vi "ScanHarmonics Nov21-2018.vi"() -> ()   [LabVIEW 2016]
uses:
  <vilib>/Instr/_visa.llb/VISA Configure Serial Port (Instr).vi
panel:
  out "Current Position 2":string="0\r\n"
  out "Start Time":string
  out "RoiSum":dbl=24008.0
  in  "Main UI":T1(tab)=enum."Collect Data"
  in  "Get Position":bool
  in  "Set Zero Position":bool
  in  "Move to Target":bool
  in  "Arduino USB Port":refnum<visa-resource-name>="COM3"
  in  "Target Motor Position":i32
  out "Current Position":string="0\r\n"
  in  "Reset Arduino":bool
  out "Settings":T2={"Range"=3520, "cftfak"=39321856, "RoiMin"=0, "RoiMax"=3520, "#Regions"=0, "Caluse"=1, "Calpoints"=0, "Param"=0, "Offset"=0, "Xdim"=0, "bitshift"=0, "Active"=1, "Roipreset"=10.0, "dummy1"=0.0, "dummy2"=0.0, "dummy3"=0.0} {"dummy3" format="%.2f"; "dummy2" format="%.2f"; "bitshift" format="%.0x"; "Active" format="%.0x"; "Offset" format="%.0x"; "Param" format="%.0x"; "dummy1" format="%.2f"; "Roipreset" format="%.2f"; "cftfak" format="%.0x"}
  in  "Maximum Scan\nPosition":dbl=3000.0
  out "Harmonics":cluster{"Y":dbl[], "Y":dbl[]}[](graph)=[{"Y"=[200.0, 300.0, 400.0, 500.0, 600.0, 700.0, 800.0, 900.0, 1000.0, 1100.0, 1200.0, 1300.0, 1400.0, 1500.0, 1600.0, 1700.0, 1800.0, 1900.0, 2000.0, 2100.0, 2200.0, 2300.0, 2400.0, 2500.0, 2600.0, 2700.0, 2800.0, 2900.0, 3000.0, 3100.0, 3200.0, 3300.0], "Y"=[0.0, 24008.0, 24008.0, 24008.0, 24008.0, 24008.0, 24008.0, 24008.0, 24008.0, 24008.0, 24008.0, 24008.0, 24008.0, 24008.0, 24008.0, 24008.0, 24008.0, 24008.0, 24008.0, 24008.0, 24008.0, 24008.0, 24008.0, 24008.0, 24008.0, 24008.0, 24008.0, 24008.0, 24008.0, 24008.0, 24008.0, 24008.0]}]
  in  "Start Scan":bool
  out "Spectrum":u32[](graph)
  in  "State":T3(ring)=enum."Move Grating"
  out "Grating Position":i16=3300
  in  "Step Size":i32=100
  in  "Sweeps":i32
  out "CHN Status":T4={"Started"=0, "Maxval"=3001, "Runtime"=0.018000000000000002, "Fifo full"=0.0, "TotalSum"=24008.0, "RoiSum"=24008.0, "Roirate"=0.0, "Sweeps"=3001.0, "Starts"=3001.0, "Dummy"=0.0} {"Dummy" format="%.2f"; "Starts" format="%.2f"; "Sweeps" format="%.2f"; "Roirate" format="%.2f"; "RoiSum" format="%.2f"; "TotalSum" format="%.2f"; "Fifo full" format="%.2f"; "Runtime" format="%.2f"}
  in  "Photoelectron Spectra Destination":path=path "C:/Users/cj09d/Desktop/SpectraTest/Today"
  out "Halt Confirmation":string="OK"
  out "MCSADat Error":i32
  in  "Spectrum #":i32
  out "Arduino Response":string="1600\r\n"
  out "Sent Message":string="M003300#"
  in  "Stop":bool
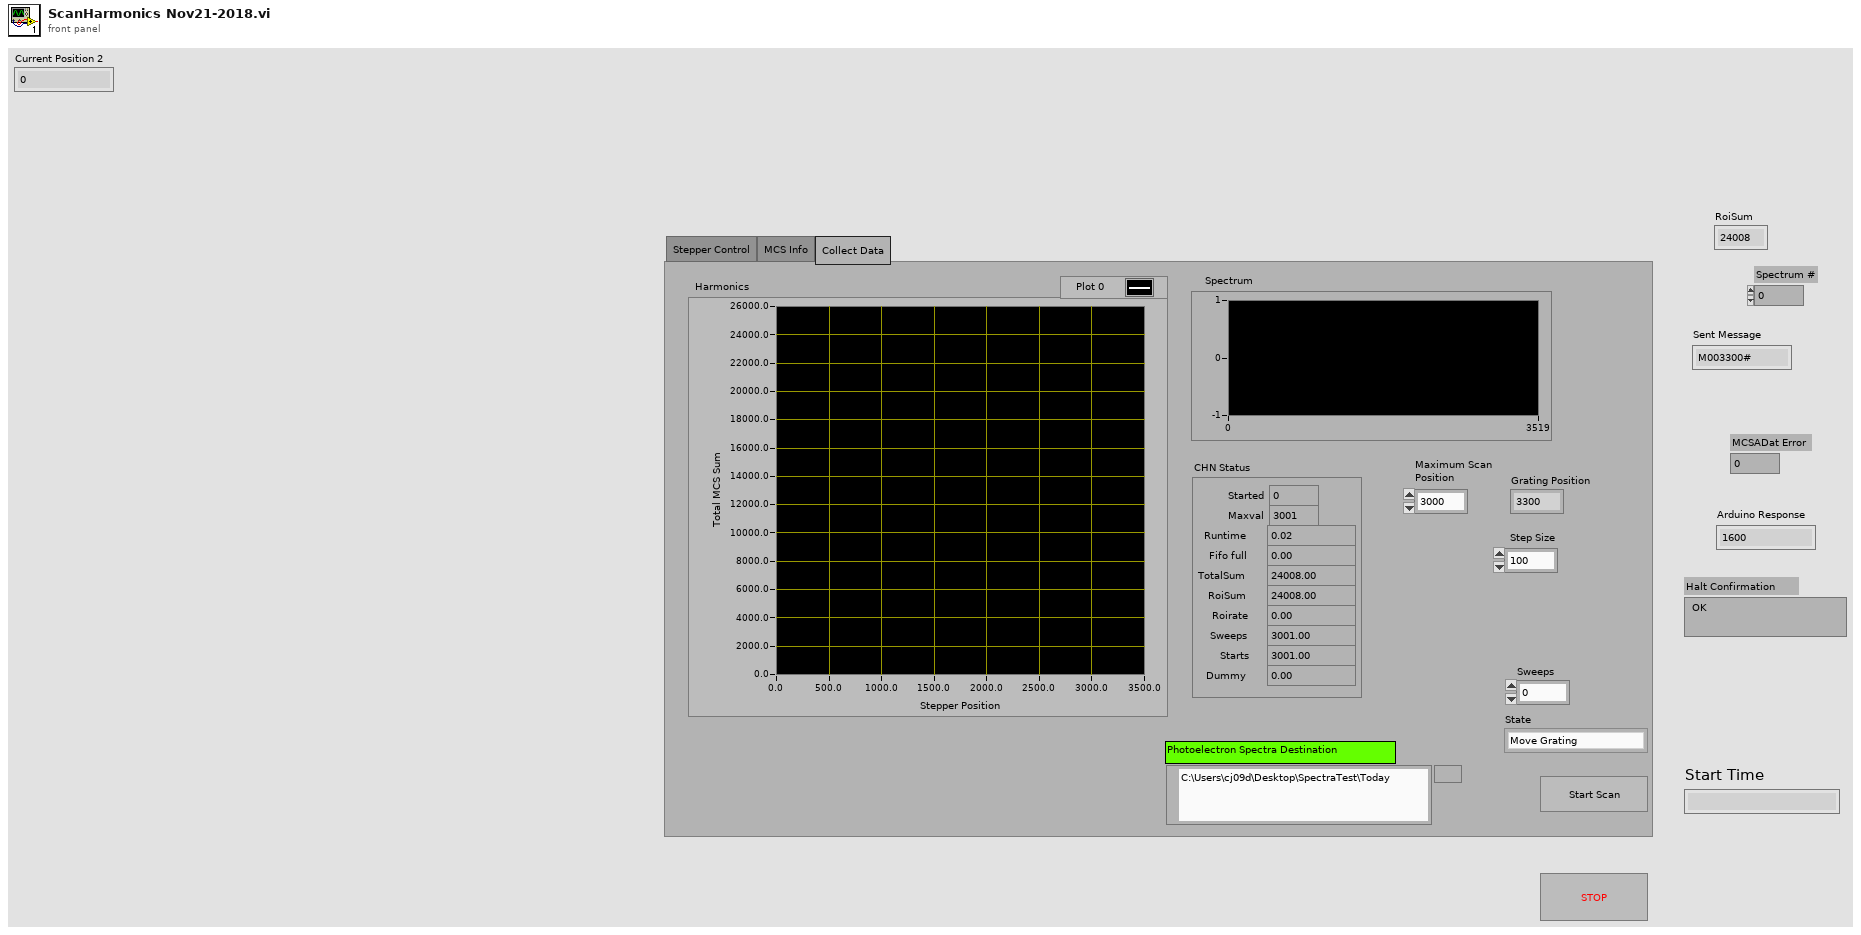
[diagram p1: front panel]
types:
  T1 = enum32{"Stepper Control", "MCS Info", "Collect Data"}
  T2 = cluster{"Range":i32, "cftfak":i32, "RoiMin":i32, "RoiMax":i32, "#Regions":i32, "Caluse":i32, "Calpoints":i32, "Param":i32, "Offset":i32, "Xdim":i32, "bitshift":i32, "Active":i32, "Roipreset":dbl, "dummy1":dbl, "dummy2":dbl, "dummy3":dbl}
  T3 = enum16{"Start", "Move Grating", "Start MCS", "Collect Data", "Stop MCS", "Save Data", "Stop"}
  T4 = cluster{"Started":i32, "Maxval":u32, "Runtime":dbl, "Fifo full":dbl, "TotalSum":dbl, "RoiSum":dbl, "Roirate":dbl, "Sweeps":dbl, "Starts":dbl, "Dummy":dbl}
  T5 = enum16{"open", "replace", "create", "open or create", "replace or create", "replace or create with confirmation"}
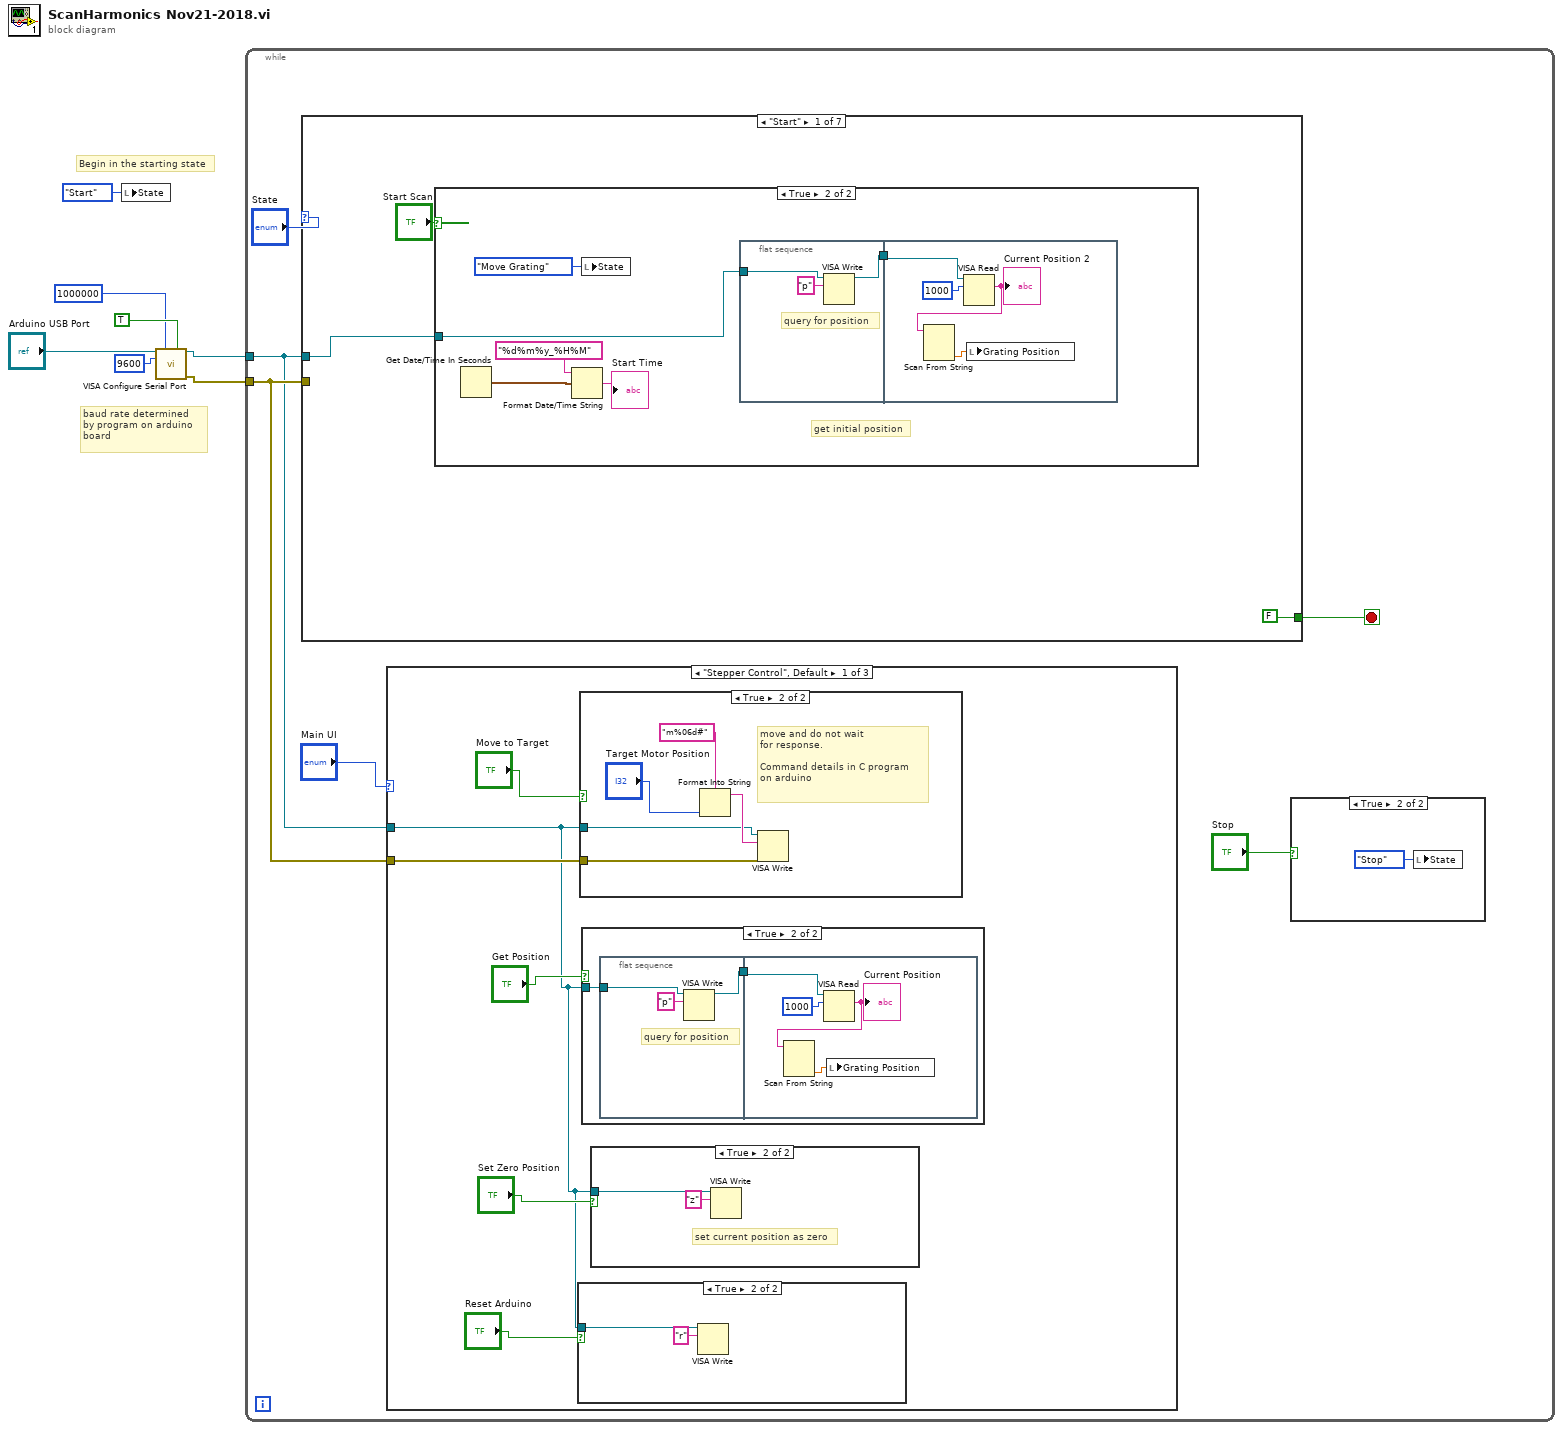
[diagram p0: block diagram]
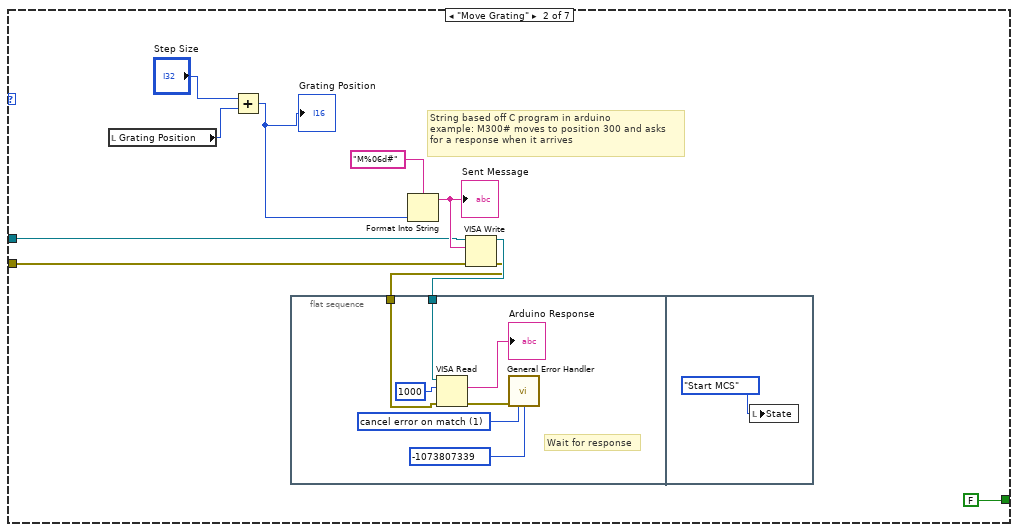
[diagram p10: hidden frame]
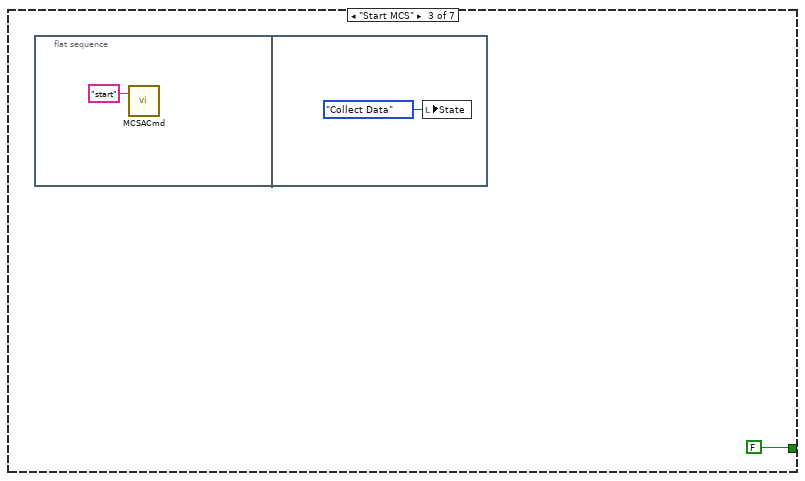
[diagram p11: hidden frame]
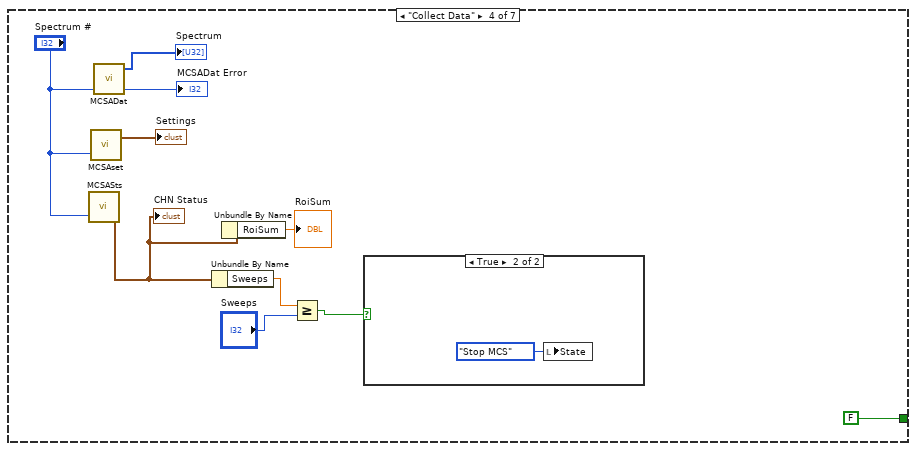
[diagram p12: hidden frame]
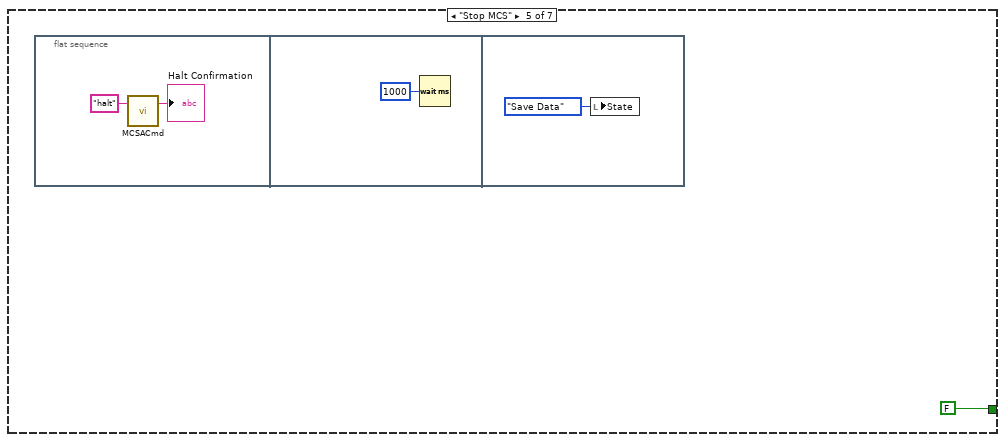
[diagram p14: hidden frame]
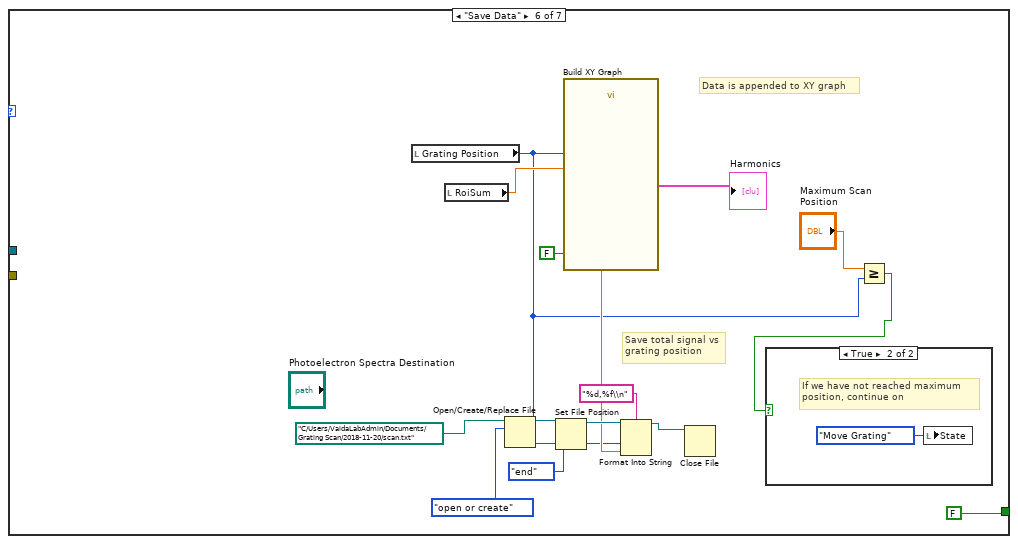
[diagram p15: hidden frame]
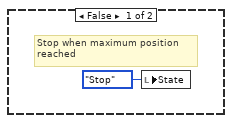
[diagram p16: hidden frame]
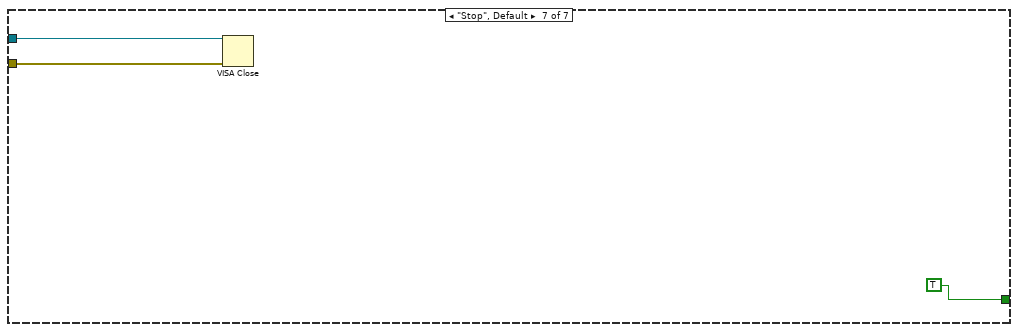
[diagram p17: hidden frame]
diagram:
  # "Begin in the starting state"
  # "baud rate determined\nby program on arduino\nboard"
  n1 = local write "State"(T3."Start" ("State")) -> ()
  n2 = call-poly "VISA Configure Serial Port"("VISA resource name"="Arduino USB Port", "timeout (10sec)"=u32 1000000, "Enable Termination\nChar (T)"=TRUE, "baud rate (9600)"=u32 9600 ("baud rate")) -> ("VISA resource name out"=w1:refnum<visa-resource-name>, "error out"=w2:errorcluster)  [unwired: 6 in, 4 out]
  n3 = while {
    tunnel: w1 -> [w10]
    tunnel: w2 -> [w11]
    stop <- w9 stop-if-true
    n4 = case shown="\"Start\"" "State" {
      tunnel: w10 -> [w39 w62 _ _ _ _ w109]
      tunnel: w11 -> [_ w61 _ _ _ _ w110]
      tunnel: [FALSE FALSE FALSE FALSE FALSE FALSE TRUE] -> w9
      frame "Start" {
        n5 = case shown="True" "Start Scan" {
          tunnel: w39 -> [_ w42]
          frame False {
          }
          frame True {
            # "get initial position"
            n6 = Get Date/Time In Seconds() -> (seconds since 1Jan1904=w45:timestamp)
            n7 = Format Date/Time String(time format string (%c)="%d%m%y_%H%M", seconds (now)=w45) -> (date/time string=→"Start Time":string)  [unwired: 1 in]
            n8 = local write "State"(T3."Move Grating" ("State")) -> ()
            n9 = flat-sequence {
              tunnel: [w50] -> w43
              tunnel: w42 -> [w48]
              tunnel: w43 -> [w53]
              frame #0 {
                # "query for position"
                n10 = VISA Write(VISA resource name=w48, write buffer="p") -> (VISA resource name out=w50:refnum<visa-resource-name>)  [unwired: 1 in, 2 out]
              }
              frame #1 {
                n11 = VISA Read(VISA resource name=w53, byte count=1000) -> (read buffer=w52:string)  [unwired: 1 in, 3 out]
                "Current Position 2" <- w52
                n12 = Scan From String(input string=w52) -> (output 1=w51:dbl)  [unwired: 4 in, 3 out]
                n13 = local write "Grating Position"(w51) -> ()
              }
            }
          }
        }
      }
      frame "Move Grating" {
        # "String based off C program in arduino\nexample: M300# moves to position 300 and asks\nfor a response when it arrives"
        n14 = local read "Grating Position"() -> (w59:i16)
        n15 = Add(x="Step Size", y=w59) -> (x+y=w56:i32)
        "Grating Position" <- w56
        n16 = flat-sequence {
          tunnel: w58 -> [w66]
          tunnel: w57 -> [w65]
          frame #0 {
            w69 = 1 items=["no exception", "cancel error on match", "set error on match"] ("[exception action] (none:0)")
            # "Wait for response"
            n17 = VISA Read(VISA resource name=w66, byte count=1000, error in (no error)=w65) -> (read buffer=→"Arduino Response":string, error out=w71:errorcluster)  [unwired: 2 out]
            n18 = call <vilib>:"General Error Handler.vi"("error in (no error)"=w71, "[exception action] (none:0)"=w69, "[exception code]"=-1073807339) -> ()  [unwired: 8 in, 5 out]
          }
          frame #1 {
            n19 = local write "State"(T3."Start MCS" ("State")) -> ()
          }
        }
        n20 = Format Into String(format string="M%06d#", w56) -> (resulting string=w63:string)  [unwired: 2 in, 1 out]
        "Sent Message" <- w63
        n21 = VISA Write(VISA resource name=w62, write buffer=w63, error in (no error)=w61) -> (VISA resource name out=w58:refnum<visa-resource-name>, error out=w57:errorcluster)  [unwired: 1 out]
      }
      frame "Start MCS" {
        n22 = flat-sequence {
          frame #0 {
            n23 = call "MCSACmd.vi"("Command"="start") -> ()  [unwired: 2 in, 1 out]
          }
          frame #1 {
            n24 = local write "State"(T3."Collect Data" ("State")) -> ()
          }
        }
      }
      frame "Collect Data" {
        n25 = call "MCSASts.vi"("CHN #"="Spectrum #") -> ("CHN Status"=w78:T4)  [unwired: 1 in, 1 out]
        "CHN Status" <- w78
        n26 = call "MCSAset.vi"("Spect #"="Spectrum #") -> ("Settings"=→"Settings":T2)  [unwired: 1 in, 1 out]
        n27 = call "MCSADat.vi"("Spectrum #"="Spectrum #") -> ("MCSADat Error"=→"MCSADat Error":i32, "Data"=→"Spectrum":u32[])  [unwired: 2 in, 1 out]
        n28 = Unbundle By Name(w78) -> ("Sweeps"=w81:dbl)
        n29 = Unbundle By Name(w78) -> ("RoiSum"=→"RoiSum":dbl)
        n30 = Greater Or Equal?(x=w81, y="Sweeps") -> (x >= y?=w79:bool)
        n31 = case shown="True" w79 {
          frame False {
            # "Do nothing, continue\ncollecting data"
          }
          frame True {
            n32 = local write "State"(T3."Stop MCS" ("State")) -> ()
          }
        }
      }
      frame "Stop MCS" {
        n33 = flat-sequence {
          frame #0 {
            n34 = call "MCSACmd.vi"("Command"="halt") -> ("Response"=→"Halt Confirmation":string)  [unwired: 2 in]
          }
          frame #1 {
            n35 = Wait (ms)(milliseconds to wait=u32 1000) -> ()  [unwired: 1 out]
          }
          frame #2 {
            n36 = local write "State"(T3."Save Data" ("State")) -> ()
          }
        }
      }
      frame "Save Data" {
        # "Data is appended to XY graph"
        # "Save total signal vs\ngrating position"
        n37 = local read "Grating Position"() -> (w95:i16)
        n38 = local read "RoiSum"() -> (w100:dbl)
        n39 = Open/Create/Replace File(file path (use dialog)=path "C:/Users/VaidaLabAdmin/Documents/Grating Scan/2018-11-20/scan.txt", operation (0:open)=T5."open or create") -> (refnum out=w103:refnum<file>)  [unwired: 4 in, 2 out]
        n40 = Set File Position(refnum=w103, from (0:start)=enum16{"start", "end", "current"}."end") -> (refnum out=w101:refnum<file>)  [unwired: 2 in, 1 out]
        n41 = call "Build XY Graph"("Reset"=FALSE, "Y Input"=w100, "X Input"=w95) -> ("XY Graph"=→"Harmonics":cluster{"X":dbl[], "Y":dbl[]}[])  [unwired: 7 in, 1 out]
        n42 = Format Into String(format string="%d,%f\\n", initial string=w101, w95, w100) -> (resulting string=w98:refnum<file>)  [unwired: 1 in, 1 out]
        n43 = Close File(refnum=w98) -> ()  [unwired: 1 in, 2 out]
        n44 = Greater Or Equal?(x="Maximum Scan\nPosition", y=w95) -> (x >= y?=w94:bool)
        n45 = case shown="True" w94 {
          frame False {
            # "Stop when maximum position\nreached"
            n46 = local write "State"(T3."Stop" ("State")) -> ()
          }
          frame True {
            # "If we have not reached maximum\nposition, continue on"
            n47 = local write "State"(T3."Move Grating" ("State")) -> ()
          }
        }
      }
      frame "Stop", Default {
        n48 = VISA Close(VISA resource name=w109, error in (no error)=w110) -> ()  [unwired: 1 out]
      }
    }
    n49 = case shown="\"Stepper Control\", Default" "Main UI" {
      tunnel: w11 -> [w18 _ _]
      tunnel: w10 -> [w15 _ _]
      frame "Stepper Control", Default {
        n50 = case shown="True" "Reset Arduino" {
          tunnel: w15 -> [_ w21]
          frame False {
          }
          frame True {
            n51 = VISA Write(VISA resource name=w21, write buffer="r") -> ()  [unwired: 1 in, 3 out]
          }
        }
        n52 = case shown="True" "Move to Target" {
          tunnel: w18 -> [_ w35]
          tunnel: w15 -> [_ w34]
          frame False {
          }
          frame True {
            # "move and do not wait\nfor response.\n\nCommand details in C program\non arduino"
            n53 = Format Into String(format string="m%06d#", "Target Motor Position") -> (resulting string=w37:string)  [unwired: 2 in, 1 out]
            n54 = VISA Write(VISA resource name=w34, write buffer=w37, error in (no error)=w35) -> ()  [unwired: 3 out]
          }
        }
        n55 = case shown="True" "Get Position" {
          tunnel: w15 -> [_ w25]
          frame False {
          }
          frame True {
            n56 = flat-sequence {
              tunnel: [w29] -> w26
              tunnel: w25 -> [w27]
              tunnel: w26 -> [w32]
              frame #0 {
                # "query for position"
                n57 = VISA Write(VISA resource name=w27, write buffer="p") -> (VISA resource name out=w29:refnum<visa-resource-name>)  [unwired: 1 in, 2 out]
              }
              frame #1 {
                n58 = VISA Read(VISA resource name=w32, byte count=1000) -> (read buffer=w31:string)  [unwired: 1 in, 3 out]
                "Current Position" <- w31
                n59 = Scan From String(input string=w31) -> (output 1=w30:dbl)  [unwired: 4 in, 3 out]
                n60 = local write "Grating Position"(w30) -> ()
              }
            }
          }
        }
        n61 = case shown="True" "Set Zero Position" {
          tunnel: w15 -> [_ w23]
          frame False {
          }
          frame True {
            # "set current position as zero"
            n62 = VISA Write(VISA resource name=w23, write buffer="z") -> ()  [unwired: 1 in, 3 out]
          }
        }
      }
      frame "MCS Info" {
        # "Ensure MCS6A.exe is running and that the 32/64 bit version of LabView matches the version of the MCS\nsoftware running, most setup done through that program\n\nIn particular set a Sweeps Preset under Hardware Options to be the desired sweeps + 1"
      }
      frame "Collect Data" {
        # "This state is continuously running based on the State variable\nSee large above case structure"
      }
    }
    n63 = case shown="True" "Stop" {
      frame False {
      }
      frame True {
        n64 = local write "State"(T3."Stop" ("State")) -> ()
      }
    }
  }
